vi "Sub00_01_ElKompilator.vi"(9 "error in (no error)":errorcluster, 10 "Enum":T1(ring), 11 "base path":path) -> (1 "error out":errorcluster)   [LabVIEW 2019]
panel:
  out "vi name":string
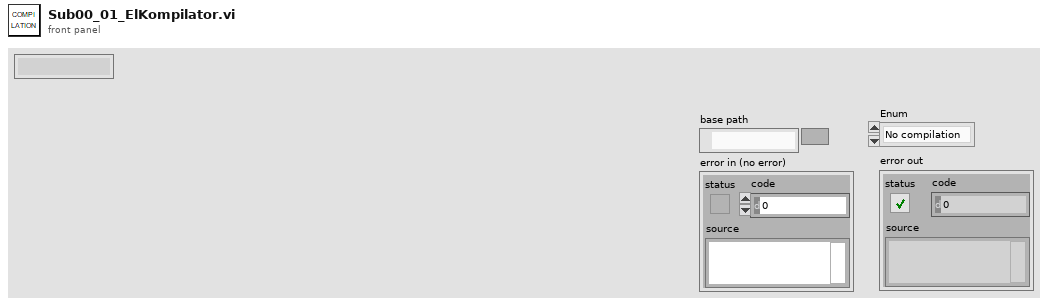
[diagram p1: front panel]
types:
  T1 = enum16{"No compilation", "No memory", "With memory", "Simple"}
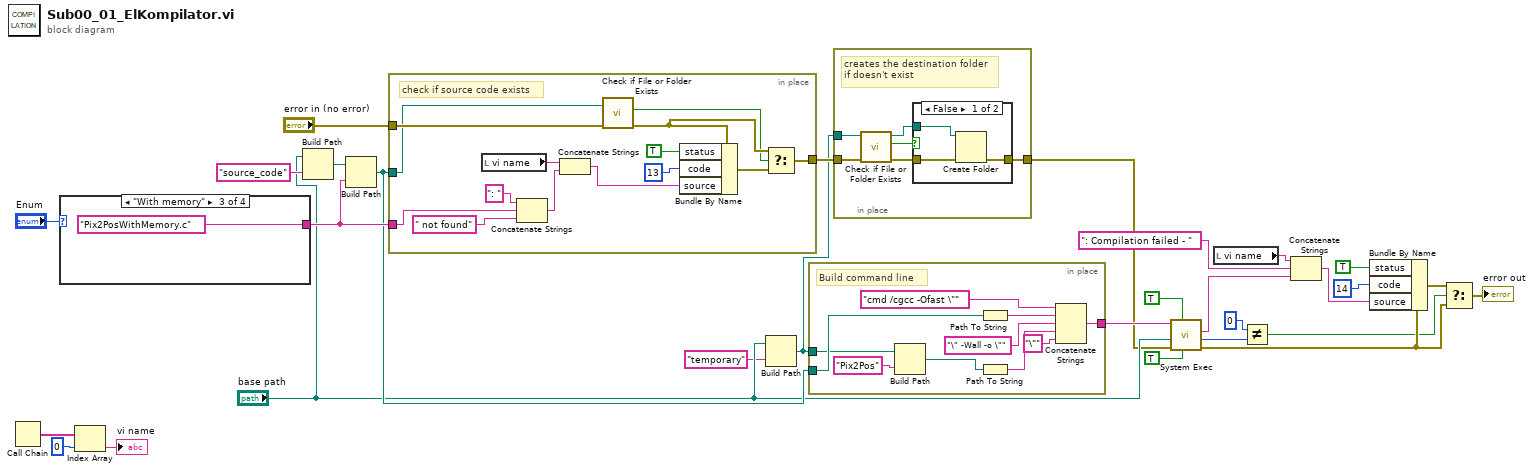
[diagram p0: block diagram]
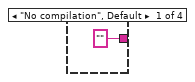
[diagram p3: hidden frame]
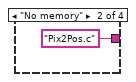
[diagram p4: hidden frame]
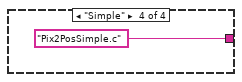
[diagram p5: hidden frame]
diagram:
  n1 = Call Chain() -> (call chain=w12:string[])
  n2 = case shown="\"With memory\"" "Enum" {
    tunnel: ["" ("name or relative path") "Pix2Pos.c" ("name or relative path") "Pix2PosWithMemory.c" ("name or relative path") "Pix2PosSimple.c" ("name or relative path")] -> w9
    frame "No compilation", Default {
    }
    frame "No memory" {
    }
    frame "With memory" {
    }
    frame "Simple" {
    }
  }
  n3 = Index Array(array=w12, index=0) -> (element=→"vi name":string)
  n4 = Build Path(base path="base path", name or relative path="source_code") -> (appended path=w28:path)
  n5 = Build Path(base path=w28, name or relative path=w9) -> (appended path=w7:path)
  n6 = in-place {
    in-place-border: w9 -> [w44]
    in-place-border: "error in (no error)" -> [w42]
    in-place-border: w7 -> [w41]
    in-place-border: [w34] -> w4
    # "check if source code exists"
    n7 = local read "vi name"() -> (w47:string)
    n8 = Concatenate Strings(": " ("string"), w44, " not found" ("string")) -> (w46:string)
    n9 = Concatenate Strings(w47, w46) -> (w36:string)
    n10 = call <vilib>:"Check if File or Folder Exists.vi"("error in (no error)"=w42, "path"=w41) -> ("error out"=w39:errorcluster, "file or folder exists?"=w35:bool)  [unwired: 7 in, 1 out]
    n11 = Bundle By Name(cluster=w39, "status"=TRUE, "code"=13, "source"=w36) -> (w40:errorcluster)
    n12 = Select(t=w39, s=w35, f=w40) -> (s? t:f=w34:errorcluster)
  }
  n13 = Build Path(base path="base path", name or relative path="temporary") -> (appended path=w1:path)
  n14 = in-place {
    in-place-border: w7 -> [w55]
    in-place-border: [w49] -> w5
    in-place-border: w1 -> [w48]
    # "Build command line"
    n15 = Build Path(base path=w48, name or relative path="Pix2Pos" ("string")) -> (appended path=w57:path)
    n16 = Path To String(path=w55) -> (string=w53:string)
    n17 = Path To String(path=w57) -> (string=w51:string)
    n18 = Concatenate Strings("cmd /cgcc -Ofast \"" ("string"), w53, "\" -Wall -o \"" ("string"), w51, "\"" ("string")) -> (w49:string)
  }
  n19 = in-place {
    in-place-border: w4 -> [w63]
    in-place-border: w1 -> [w62]
    in-place-border: [w58] -> w3
    # "creates the destination folder\nif doesn't exist"
    n20 = call <vilib>:"Check if File or Folder Exists.vi"("error in (no error)"=w63, "path"=w62) -> ("error out"=w60:errorcluster, "file or folder exists?"=w61:bool, "dup path"=w59:path)  [unwired: 7 in]
    n21 = case shown="False" w61 {
      tunnel: w60 -> [w66 w67]
      tunnel: w59 -> [w65 _]
      tunnel: [w64 w67] -> w58
      frame False {
        n22 = Create Folder(path (use dialog)=w65, error in=w66) -> (error out=w64:errorcluster)  [unwired: 1 in, 2 out]
      }
      frame True {
      }
    }
  }
  n23 = call <vilib>:"System Exec.vi"("run minimized? (F)"=TRUE, "wait until completion? (T)"=TRUE, "error in (no error)"=w3, "working directory"="base path", "command line"=w5) -> ("error out"=w23:errorcluster, "return code"=w21:i32, "standard error"=w27:string)  [unwired: 3 in, 1 out]
  n24 = local read "vi name"() -> (w26:string)
  n25 = Not Equal?(x=0 ("y"), y=w21) -> (x != y?=w22:bool)
  n26 = Concatenate Strings(w26, ": Compilation failed - " ("string"), w27) -> (w24:string)
  n27 = Bundle By Name(cluster=w23, "status"=TRUE, "code"=14, "source"=w24) -> (w25:errorcluster)
  n28 = Select(t=w25, s=w22, f=w23) -> (s? t:f=→"error out":errorcluster)
